vi "Drive Sideways.vi"(1 "Setpoint":dbl) -> ()   [LabVIEW 2017]
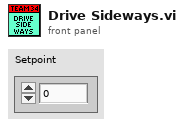
[diagram p1: front panel]
types:
  T1 = typedef "WPI_EncoderDevRef.ctl" = cluster{"DevStatus":errorcluster, "EncoderIndex":T2, "CounterIndex":T3, "DistancePerCount":dbl, "Decoding Type":T4}
  T2 = typedef "FPGA_EncoderIdx.ctl" = enum8{"Enc 0", "Enc 1", "Enc 2", "Enc 3", "Enc 4", "Enc 5", "Enc 6", "Enc 7", "Invalid"}
  T3 = typedef "FPGA_CounterCtrSystemIndex.ctl" = enum8{"Ctr 0", "Ctr 1", "Ctr 2", "Ctr 3", "Ctr 4", "Ctr 5", "Ctr 6", "Ctr 7", "Invalid"}
  T4 = typedef "WPI_EncoderType.ctl" = enum16{"1x", "2x", "4x"}
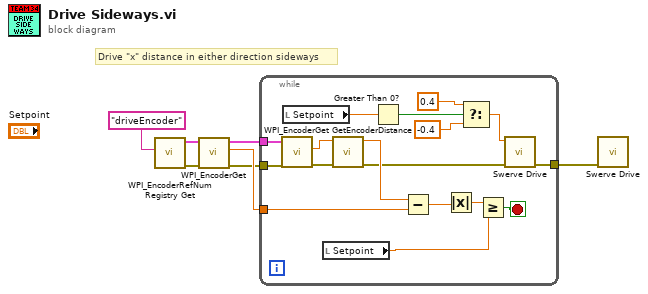
[diagram p0: block diagram]
diagram:
  # "Drive \"x\" distance in either direction sideways"
  n1 = call <vilib>:"WPI_EncoderRefNum Registry Get.vi"("refnum name"="driveEncoder") -> ("error out"=w1:errorcluster, "EncoderDevRef"=w2:T1)  [unwired: 9 in]
  n2 = call <vilib>:"WPI_EncoderGet.vi"("error in (no error)"=w1, "EncoderDevRef"=w2) -> ("error out"=w4:errorcluster, "Distance"=w6:dbl, "EncoderDevRef"=w5:T1)  [unwired: 4 in, 3 out]
  n3 = while {
    tunnel: w4 -> [w24]
    tunnel: w5 -> [w23]
    tunnel: w6 -> [w22]
    tunnel: [w18] -> w7
    stop <- w19 stop-if-true
    n4 = call <vilib>:"WPI_EncoderGet.vi"("error in (no error)"=w24, "EncoderDevRef"=w23) -> ("error out"=w12:errorcluster, "Distance"=w14:dbl)  [unwired: 4 in, 4 out]
    n5 = local read "Setpoint"() -> (w8:dbl)
    n6 = local read "Setpoint"() -> (w9:dbl)
    n7 = call "GetEncoderDistance.vi"("Error In"=w12, "Distance"=w14) -> ("Error Out"=w11:errorcluster, "Distance Travelled (in)"=w13:dbl)  [unwired: 8 in]
    n8 = Greater Than 0?(x=w8) -> (x > 0?=w17:bool)
    n9 = Subtract(x=w13, y=w22) -> (x-y=w21:dbl)
    n10 = Absolute Value(x=w21) -> (abs(x)=w20:dbl)
    n11 = Select(t=0.4, s=w17, f=-0.4) -> (s? t:f=w10:dbl)
    n12 = Greater Or Equal?(x=w20, y=w9) -> (x >= y?=w19:bool)
    n13 = call "Swerve Drive.vi"("X"=w10, "Error In"=w11) -> ("Error Out"=w18:errorcluster)  [unwired: 9 in, 4 out]
  }
  n14 = call "Swerve Drive.vi"("Error In"=w7) -> ()  [unwired: 10 in, 5 out]
